vi "CANrangeGetters.vi"   [LabVIEW 2023]
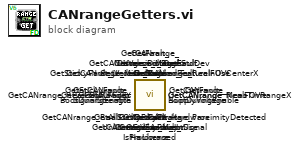
[diagram p0: block diagram]
diagram:
  n1 = call <vilib>:"GetStickyFault_UnlicensedFeatureInUse.vi"() -> ()  [unwired: 10 in, 2 out]
  n2 = call <vilib>:"GetFault_UnlicensedFeatureInUse.vi"() -> ()  [unwired: 10 in, 2 out]
  n3 = call <vilib>:"GetStickyFault_BootDuringEnable.vi"() -> ()  [unwired: 10 in, 2 out]
  n4 = call <vilib>:"GetFault_BootDuringEnable.vi"() -> ()  [unwired: 10 in, 2 out]
  n5 = call <vilib>:"GetStickyFault_Undervoltage.vi"() -> ()  [unwired: 10 in, 2 out]
  n6 = call <vilib>:"GetFault_Undervoltage.vi"() -> ()  [unwired: 10 in, 2 out]
  n7 = call <vilib>:"GetStickyFault_Hardware.vi"() -> ()  [unwired: 10 in, 2 out]
  n8 = call <vilib>:"GetFault_Hardware.vi"() -> ()  [unwired: 10 in, 2 out]
  n9 = call <vilib>:"GetCANrange_RealFOVRangeY.vi"() -> ()  [unwired: 10 in, 2 out]
  n10 = call <vilib>:"GetCANrange_RealFOVRangeX.vi"() -> ()  [unwired: 10 in, 2 out]
  n11 = call <vilib>:"GetCANrange_RealFOVCenterY.vi"() -> ()  [unwired: 10 in, 2 out]
  n12 = call <vilib>:"GetCANrange_RealFOVCenterX.vi"() -> ()  [unwired: 10 in, 2 out]
  n13 = call <vilib>:"GetCANrange_DistanceStdDev.vi"() -> ()  [unwired: 10 in, 2 out]
  n14 = call <vilib>:"GetCANrange_AmbientSignal.vi"() -> ()  [unwired: 10 in, 2 out]
  n15 = call <vilib>:"GetCANrange_MeasState.vi"() -> ()  [unwired: 10 in, 2 out]
  n16 = call <vilib>:"GetCANrange_ProximityDetected.vi"() -> ()  [unwired: 10 in, 2 out]
  n17 = call <vilib>:"GetCANrange_SignalStrength.vi"() -> ()  [unwired: 10 in, 2 out]
  n18 = call <vilib>:"GetCANrange_MeasTime.vi"() -> ()  [unwired: 10 in, 2 out]
  n19 = call <vilib>:"GetCANrange_Distance_Meters.vi"() -> ()  [unwired: 10 in, 2 out]
  n20 = call <vilib>:"GetCANrange_SupplyVoltage.vi"() -> ()  [unwired: 10 in, 2 out]
  n21 = call <vilib>:"GetVersion_IsProLicensed.vi"() -> ()  [unwired: 10 in, 2 out]
  n22 = call <vilib>:"GetAllStickyFaults.vi"() -> ()  [unwired: 10 in, 2 out]
  n23 = call <vilib>:"GetAllFaults.vi"() -> ()  [unwired: 10 in, 2 out]
  n24 = call <vilib>:"GetVersion_Full.vi"() -> ()  [unwired: 10 in, 2 out]
  n25 = call <vilib>:"GetVersion_Build.vi"() -> ()  [unwired: 10 in, 2 out]
  n26 = call <vilib>:"GetVersion_Bugfix.vi"() -> ()  [unwired: 10 in, 2 out]
  n27 = call <vilib>:"GetVersion_Minor.vi"() -> ()  [unwired: 10 in, 2 out]
  n28 = call <vilib>:"GetVersion_Major.vi"() -> ()  [unwired: 10 in, 2 out]
